vi "Pot Volt converter.vi"(6 "Convert to Degrees?":bool, 8 "Pot range from center (Degrees)":dbl=90.0, 9 "Pot Max":dbl=5.0, 10 "Pot Midpoint":dbl=2.5, 11 "Pot In":dbl) -> (2 "Pot Out":dbl)   [LabVIEW 2011]
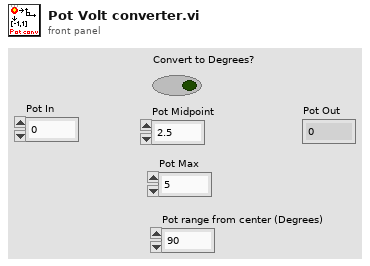
[diagram p1: front panel]
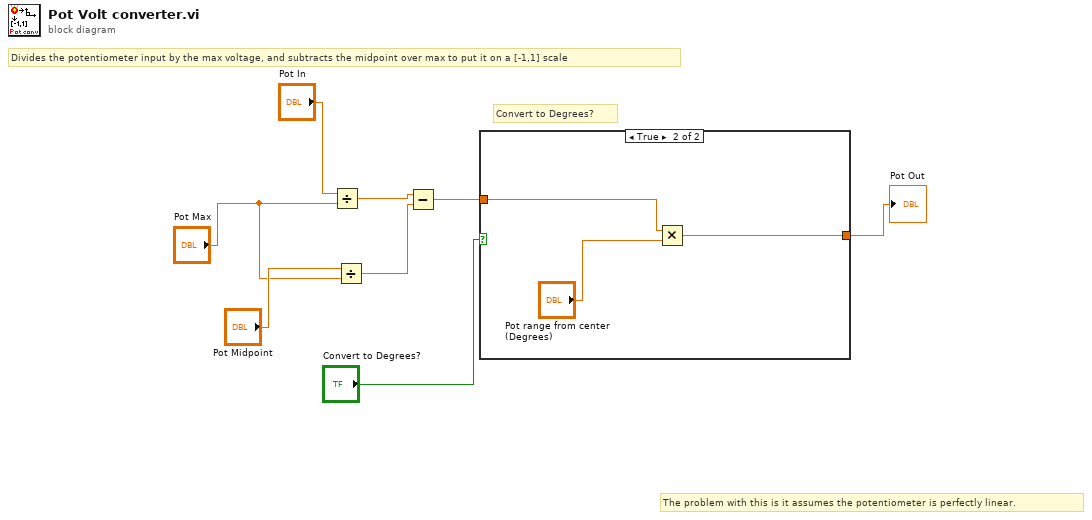
[diagram p0: block diagram]
diagram:
  # "The problem with this is it assumes the potentiometer is perfectly linear."
  # "Convert to Degrees?"
  # "Divides the potentiometer input by the max voltage, and subtracts the midpoint over max to put it on a [-1,1] scale"
  n1 = Divide(x="Pot In", y="Pot Max") -> (x/y=w7:dbl)
  n2 = Divide(x="Pot Midpoint", y="Pot Max") -> (x/y=w4:dbl)
  n3 = Subtract(x=w7, y=w4) -> (x-y=w2:dbl)
  n4 = case shown="True" "Convert to Degrees?" {
    tunnel: w2 -> [w9 w11]
    tunnel: [w9 w10] -> w1
    frame False {
    }
    frame True {
      n5 = Multiply(x=w11, y="Pot range from center (Degrees)") -> (x*y=w10:dbl)
    }
  }
  "Pot Out" <- w1
